vi "New CAP1208 Device.vi"(8 "error in (no error)":errorcluster, 10 "I2C Slave Address (0x28)":u8=40 format="%.0x", 11 "I2C":refnum<class "LINX I2C.lvclass">) -> (0 "error out":errorcluster, 3 "CAP1208 out":refnum<class "CAP1208.lvclass">)   [LabVIEW 2020, in "CAP1208.lvclass"]
uses:
  CAP1208.lvclass
  LINX I2C/LINX I2C.lvclass
  CAP1208.lvclass/CAP1208.ctl
  Write I2C.vi
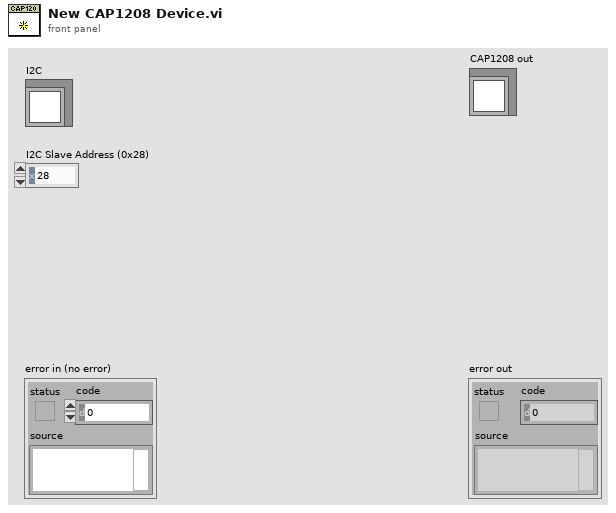
[diagram p1: front panel]
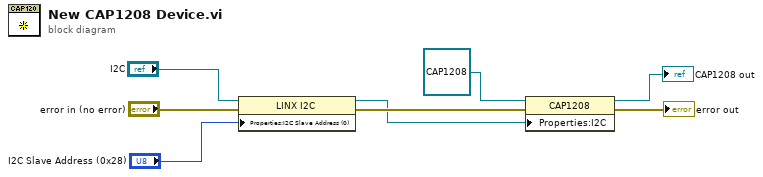
[diagram p0: block diagram]
diagram:
  n1 = property class="LINX I2C"(reference="I2C", error in="error in (no error)", "Properties:I2C Slave Address (0)"="I2C Slave Address (0x28)") -> (reference out=w3:refnum<class "LINX I2C.lvclass">, error out=w4:errorcluster)
  n2 = property class="CAP1208"(reference=refnum<class "CAP1208.lvclass"> refnum ("CAP1208 in"), error in=w4, "Properties:I2C"=w3) -> (reference out=→"CAP1208 out":refnum<class "CAP1208.lvclass">, error out=→"error out":errorcluster)
